vi "Extract Single Tone Information N Chan (CDB).vi"(6 "advanced search":T1={"approx freq. (optional)"=nan, "search (+/- % of Fsampl.)"=5.0} {"search (+/- % of Fsampl.)" format="%0.2p"; "approx freq. (optional)" format="%0.2p"}, 8 "error in (no error)":errorcluster, 10 "export mode":T2(ring), 11 "time signals in":waveform(cdb)[](array[waveform])) -> (0 "error out":errorcluster, 1 "detected phases (deg)":dbl[](array[numeric]) format="%.2p", 2 "detected amplitudes":dbl[](array[numeric]) format="%.2p", 3 "detected frequencies":dbl[](array[numeric]) format="%.2p", 4 "measurements info":T3(array[cluster]) {"uncertainty" format="%0.2p"}, 5 "exported signals":T4(array[cluster]) {"exported spectrum (dB)"."dB Spectrum (Hann)" format="%.2p"; "exported spectrum (dB)"."df" format="%.2p"; "exported spectrum (dB)"."f0" format="%.2p"})   [LabVIEW 2020, in "NI_MAPro.lvlib"]
doc: "Takes a signal in, finds the single tone with the highest amplitude or searches a specified frequency range, and returns the single tone frequency, amplitude, and phase. The input signal can be real or complex and single-channel or multichannel. Wire data to the <B>time signal in</B> input to determine the polymorphic instance to use or manually select the instance."
uses:
  NI_MAPro.lvlib
  NI_MABase.lvlib
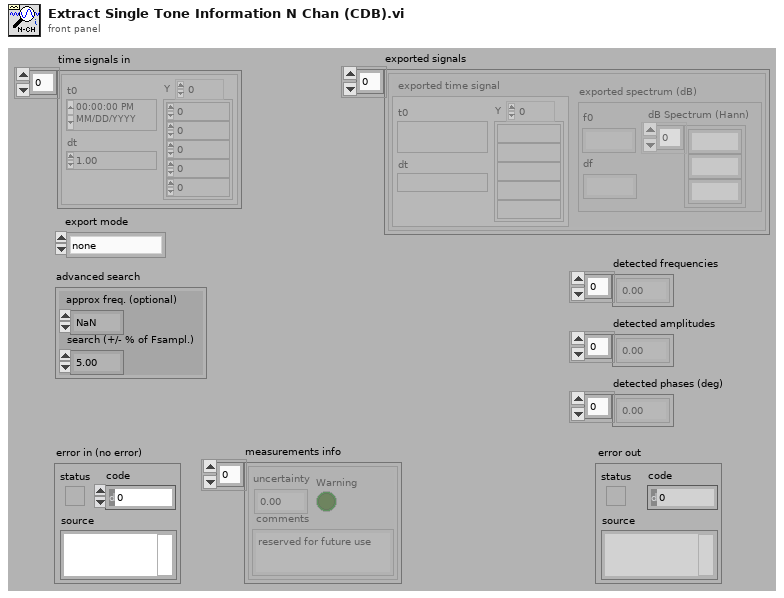
[diagram p1: front panel]
types:
  T1 = cluster{"approx freq. (optional)":dbl, "search (+/- % of Fsampl.)":dbl}
  T2 = enum32{"none", "input signal", "detected signal", "residual signal"}
  T3 = cluster{"uncertainty":dbl, "Warning":bool, "comments":string}[]
  T4 = cluster{"exported time signal":waveform(cdb), "exported spectrum (dB)":cluster{"f0":dbl, "df":dbl, "dB Spectrum (Hann)":dbl[]}}[]
  T5 = cluster{"uncertainty":dbl, "Warning":bool, "comments":string}
  T6 = cluster{"exported time signal":waveform(cdb), "exported spectrum (dB)":cluster{"f0":dbl, "df":dbl, "dB Spectrum (Hann)":dbl[]}}
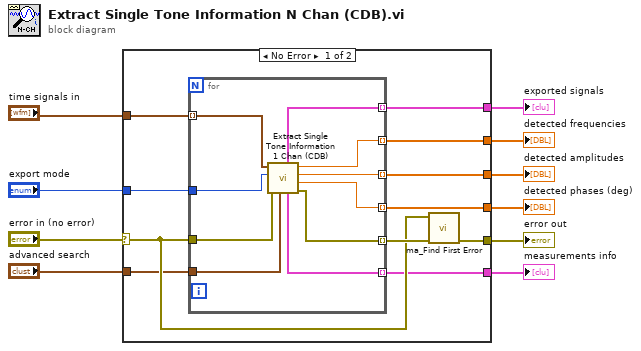
[diagram p0: block diagram]
diagram:
  n1 = case shown="No Error" "error in (no error)" {
    selector: "error in (no error)" -> [w19 w32]
    tunnel: [w20 w32] -> w9
    tunnel: [w18 _] -> w8
    tunnel: [w17 _] -> w7
    tunnel: [w16 _] -> w6
    tunnel: [w15 _] -> w5
    tunnel: [w14 _] -> w4
    tunnel: "export mode" -> [w13 _]
    tunnel: "time signals in" -> [w12 _]
    tunnel: "advanced search" -> [w11 _]
    frame No Error {
      n2 = for {
        tunnel: w11 -> [w27]
        tunnel: [w25] -> w16 mode=indexing
        tunnel: [w24] -> w15 mode=indexing
        tunnel: [w23] -> w14 mode=indexing
        tunnel: w13 -> [w30]
        tunnel: w12 -> [w31] mode=indexing
        tunnel: [w26] -> w17 mode=indexing
        tunnel: w19 -> [w29]
        tunnel: [w28] -> w21 mode=indexing
        tunnel: [w22] -> w18 mode=indexing
        n3 = call "Extract Single Tone Information 1 Chan (CDB).vi"("advanced search"=w27, "error in (no error)"=w29, "export mode"=w30, "time signal in"=w31) -> ("error out"=w28:errorcluster, "detected phase (deg)"=w23:dbl, "detected amplitude"=w24:dbl, "detected frequency"=w25:dbl, "measurement info"=w22:T5, "exported signals"=w26:T6)  [unwired: 2 out]
      }
      n4 = call "ma_Find First Error.vi"("error array in"=w21, "error in 1 (no error)"=w19) -> ("error out"=w20:errorcluster)  [unwired: 2 in, 3 out]
    }
    frame Error {
    }
  }
  "error out" <- w9
  "measurements info" <- w8
  "detected phases (deg)" <- w4
  "detected frequencies" <- w6
  "detected amplitudes" <- w5
  "exported signals" <- w7
